vi "Demo2 (Host).vi"() -> ()   [LabVIEW 2023]
uses:
  <vilib>/rvi/interface/nirviOpenFPGA/nirviOpenFPGA.xnode
  <vilib>/rvi/interface/nirviMethod/nirviMethod.xnode
  <vilib>/rvi/interface/nirviCloseFPGA/nirviCloseFPGA.xnode
  <vilib>/addons/Digital Filter Design/NI_DigFilterLicensed.lvlib
  <vilib>/addons/Digital Filter Design/FXPSim.llb/DFD FXP Postprocessing (I16, nCh).vi
  <vilib>/addons/Digital Filter Design/FilterLib.llb/DFD Load Filter from File.vi
  <vilib>/rvi/errors/niLvFpgaMergeErrorWithErrorCode.vi
  FPGA Bitfiles/Demo2_DFDTFilterTarget_Demo2(FPGA)_hKmL+IvS8gY.lvbitx
  Demo2 (FPGA).vi
  <vilib>/userdefined/High Color/nirio_resource_hc.ctl
panel:
  in  "resource name":T1
  in  "stop":bool
  out "Filtered Signal":dbl[][](graph)
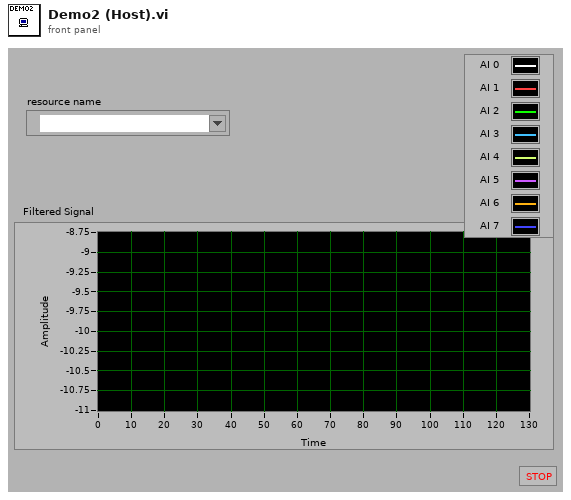
[diagram p1: front panel]
types:
  T1 = typedef "nirio_resource_hc.ctl" = tag
  T2 = typedef "NI_DigFilterLicensed.lvlib/DFD Filter Obj.ctl" = cluster{"mSRate_Fs":dbl, "mSRate_Version":string, "mSRate_Comments":string, "mSRate_OrgCoef":T3, "mSRate_CurCoef":T3, "mSRate_Quantized?":bool, "mSRate_QCoef":T3, "mSRate_QSettings":T5[], "mSRate_Order":i32, "mSRate_Scaling":cluster{"mSRate_ScaleByPowerOf2?":bool, "mSRate_ScaleType":T7}}
  T3 = typedef "NI_DigFilterLicensed.lvlib/DFD Filter Coef.ctl" = cluster{"type":T4, "gain":dbl, "coef a (k)":dbl[], "coef b (v)":dbl[]}
  T4 = typedef "NI_DigFilterLicensed.lvlib/DFD Filter Structure Type Selector.ctl" = enum16{"Undefined", "FIR Direct Form", "FIR Direct Form Transposed", "FIR Symmetric", "FIR Antisymmetric", "IIR Direct Form I", "IIR Direct Form I Transposed", "IIR Direct Form II", "IIR Direct Form II Transposed", "IIR Cascaded Second Order Sections Form I", "IIR Cascaded Second Order Sections Form I Transposed", "IIR Cascaded Second Order Sections Form II", "IIR Cascaded Second Order Sections Form II Transposed", "Lattice Allpass (basic sections)", "Lattice Allpass (one multiplier sections)", "Lattice Allpass (normalized sections)", "Lattice AR (basic sections)", "Lattice AR (one multiplier sections)", "Lattice AR (normalized sections)", "Lattice MA (minimum phase)", "Lattice MA (maximum phase)", "Lattice ARMA (basic sections)", "Lattice ARMA (one multiplier sections)", "Lattice ARMA (normalized sections)"}
  T5 = typedef "NI_DigFilterLicensed.lvlib/dfd_Internal Quantization Settings.ctl" = cluster{"source":T6, "wl":i16, "iwl":i16, "overflow mode":enum16{"Saturation", "Wrap"}, "rounding mode":enum16{"Nearest", "Truncation"}, "signed?":bool}
  T6 = typedef "NI_DigFilterLicensed.lvlib/dfd_Internal Quantization Srcs.ctl" = u16
  T7 = typedef "NI_DigFilterLicensed.lvlib/DFD Coef Norm Type.ctl" = enum16{"No Norm", "Time Domain 1-Norm", "Time Domain 2-Norm", "Time Domain Inf-Norm"}
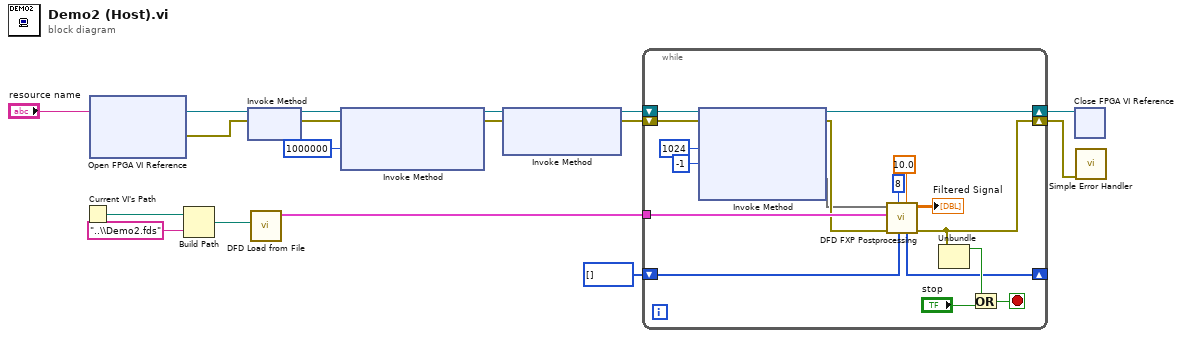
[diagram p0: block diagram]
diagram:
  n1 = Current VI's Path() -> (path=w5:path)
  n2 = xnode "Open FPGA VI Reference"("resource name"="resource name") -> ("FPGA VI Reference Out"=w17:refnum<k20>, "error out"=w16:errorcluster)  [unwired: 1 in]
  n3 = Build Path(base path=w5, name or relative path="..\\Demo2.fds") -> (appended path=w3:path)
  n4 = xnode "Invoke Method"("FPGA VI Reference In"=w17, "error in"=w16) -> ("FPGA VI Reference Out"=w15:refnum<k20>, "error out"=w14:errorcluster)
  n5 = call-poly <vilib>:"DFD Load from File.vi"("file path in"=w3) -> ("filter out"=w2:T2)  [unwired: 1 in, 9 out]
  n6 = xnode "Invoke Method"("FPGA VI Reference In"=w15, "error in"=w14, "Requested Depth"=u32 1000000 ("Depth")) -> ("FPGA VI Reference Out"=w12:refnum<k20>, "error out"=w11:errorcluster)  [unwired: 1 out]
  n7 = xnode "Invoke Method"("FPGA VI Reference In"=w12, "error in"=w11) -> ("FPGA VI Reference Out"=w10:refnum<k20>, "error out"=w9:errorcluster)  [unwired: 1 in]
  n8 = while {
    shift-right: [w25] -> w7
    shift-left: w9 -> [w33]
    tunnel: w2 -> [w30]
    shift-right: [w26] -> w8
    shift-left: w10 -> [w34]
    shift-right: [w20] -> _
    shift-left: i16[] [] ("history out") -> [w19]
    stop <- w22 stop-if-true
    n9 = xnode "Invoke Method"("FPGA VI Reference In"=w34, "error in"=w33, "Number of Elements"=u32 1024, "Timeout (ms)"=-1) -> ("FPGA VI Reference Out"=w26:refnum<k20>, "error out"=w29:errorcluster, "Data"=w18:void[])  [unwired: 1 out]
    n10 = call-poly <vilib>:"DFD FXP Postprocessing.vi"("input range"=10.0, "history in"=w19, "# channels"=8, "error in (no error)"=w29, "filter"=w30, "signal in"=w18) -> ("error out"=w25:errorcluster, "signal out"=→"Filtered Signal":dbl[][], "history out"=w20:i16[])  [unwired: 3 out]
    n11 = Unbundle(w25) -> ("status"=w23:bool)  [unwired: 2 out]
    n12 = Or(x=w23, y="stop") -> (x .or. y?=w22:bool)
  }
  n13 = xnode "Close FPGA VI Reference"("FPGA VI Reference In"=w8) -> ()  [unwired: 1 in, 1 out]
  n14 = call <vilib>:"Simple Error Handler.vi"("error in (no error)"=w7) -> ()  [unwired: 1 in, 8 out]
